vi "log_sampling.vi"(9 "q_samples":i32=100, 10 "stop_us":dbl=300.0 min=0.01, 11 "start_us":dbl=0.01 min=0.01) -> (2 "min_step_us":dbl format="%.5f", 3 "sampling_times_us":dbl[](array[numeric]))   [LabVIEW 2018]
uses:
  <vilib>/Analysis/1siggen.llb/Ramp Pattern by Samples.vi
  <vilib>/Analysis/NI_AALBase.lvlib
panel:
  out "coerced_times_us":dbl[](array[numeric])
  out "log_samples_us":dbl[](array[numeric])
  # "-"
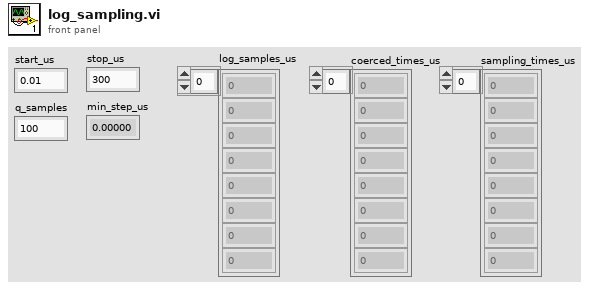
[diagram p1: front panel]
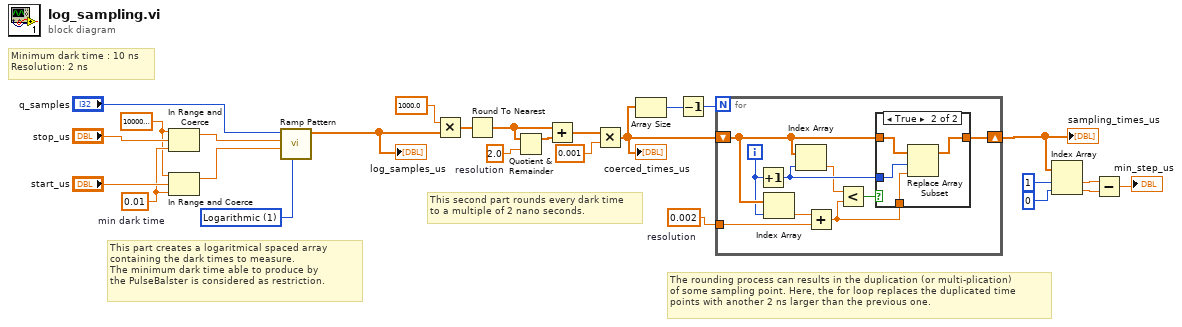
[diagram p0: block diagram]
diagram:
  w5 = 0.002  # resolution
  w13 = 2.0  # resolution
  w15 = 10000000.0 ("upper limit")
  w16 = 0.01  # min dark time
  w26 = u16 1 items=["Linear", "Logarithmic"] ("type")
  # "The rounding process can results in the duplication (or multi-plication)\nof some sampling point. Here, the for loop replaces the duplicated time \npoints with another 2 ns larger than the previous one."
  # "This second part rounds every dark time\nto a multiple of 2 nano seconds."
  # "This part creates a logaritmical spaced array\ncontaining the dark times to measure.\nThe minimum dark time able to produce by\nthe PulseBalster is considered as restriction."
  # "Minimum dark time : 10 ns\nResolution: 2 ns"
  n1 = In Range and Coerce(upper limit=w15, x="stop_us", lower limit=w16) -> (coerced(x)=w18:dbl)  [unwired: 1 out]
  n2 = In Range and Coerce(upper limit=w15, x="start_us", lower limit=w16) -> (coerced(x)=w19:dbl)  [unwired: 1 out]
  n3 = call-poly <vilib>:"Ramp Pattern.vi"("type"=w26, "start"=w19, "end"=w18, "samples"="q_samples") -> ("Ramp Pattern"=w7:dbl[])  [unwired: 6 in, 1 out]
  "log_samples_us" <- w7
  n4 = Multiply(x=1000.0 ("y"), y=w7) -> (x*y=w14:dbl[])
  n5 = Round To Nearest(number=w14) -> (nearest integer value=w11:dbl[])
  n6 = Quotient & Remainder(x=w11, y=w13) -> (x-y*floor(x/y)=w12:dbl[])  [unwired: 1 out]
  n7 = Add(x=w11, y=w12) -> (x+y=w9:dbl[])
  n8 = Multiply(x=w9, y=0.001) -> (x*y=w4:dbl[])
  "coerced_times_us" <- w4
  n9 = Array Size(array=w4) -> (size(s)=w2:i32)
  n10 = Decrement(x=w2) -> (x-1=w3:i32)
  n11 = for {
    N: w3 -> [_]
    shift-right: [w35] -> w1
    shift-left: w4 -> [w31]
    tunnel: w5 -> [w32]
    i -> [w29]
    n12 = Increment(x=w29) -> (x+1=w34:i32)
    n13 = Index Array(array=w31, index=w29) -> (element=w30:dbl)
    n14 = Index Array(array=w31, index=w34) -> (element=w27:dbl)
    n15 = Add(x=w30, y=w32) -> (x+y=w28:dbl)
    n16 = Less?(x=w27, y=w28) -> (x < y?=w33:bool)
    n17 = case shown="True" w33 {
      tunnel: w31 -> [w36 w40]
      tunnel: [w36 w39] -> w35
      tunnel: w34 -> [_ w38]
      tunnel: w28 -> [_ w37]
      frame False {
      }
      frame True {
        n18 = Replace Array Subset(array=w40, new element=w37, index=w38) -> (w39:dbl[])
      }
    }
  }
  "sampling_times_us" <- w1
  n19 = Index Array(array=w1, index #1=1 ("index"), index #2=0 ("index")) -> (element #1=w22:dbl, element #2=w21:dbl)
  n20 = Subtract(x=w22, y=w21) -> (x-y=→"min_step_us":dbl)
